vi "Get Arm Sensor Info.vi"(5 "error in (no error)":errorcluster, 6 "MotorControlDevRef":T1) -> (0 "error out":errorcluster, 1 "Current":dbl, 2 "Sensor Velocity":dbl, 3 "MotorControlDevRef out":T1, 4 "Sensor Position":dbl)   [LabVIEW 2020]
uses:
  <vilib>/Rock Robotics/WPI/MotorControl/WPI_MotorControlDeviceRef.ctl
  <vilib>/Rock Robotics/WPI/MotorControl/WPI_MotorControlType.ctl
  <vilib>/Rock Robotics/SystemInterfaces/DIO/FPGA_DIOPWMChannel.ctl
  <vilib>/Rock Robotics/WPI/PWM/WPI_PWMDeadband.ctl
  <vilib>/Rock Robotics/SystemInterfaces/DIO/FPGA_DIOChannel.ctl
  2023 Robot Global Data.vi
  <vilib>/Rock Robotics/Network Tables/NT Write Number.vi
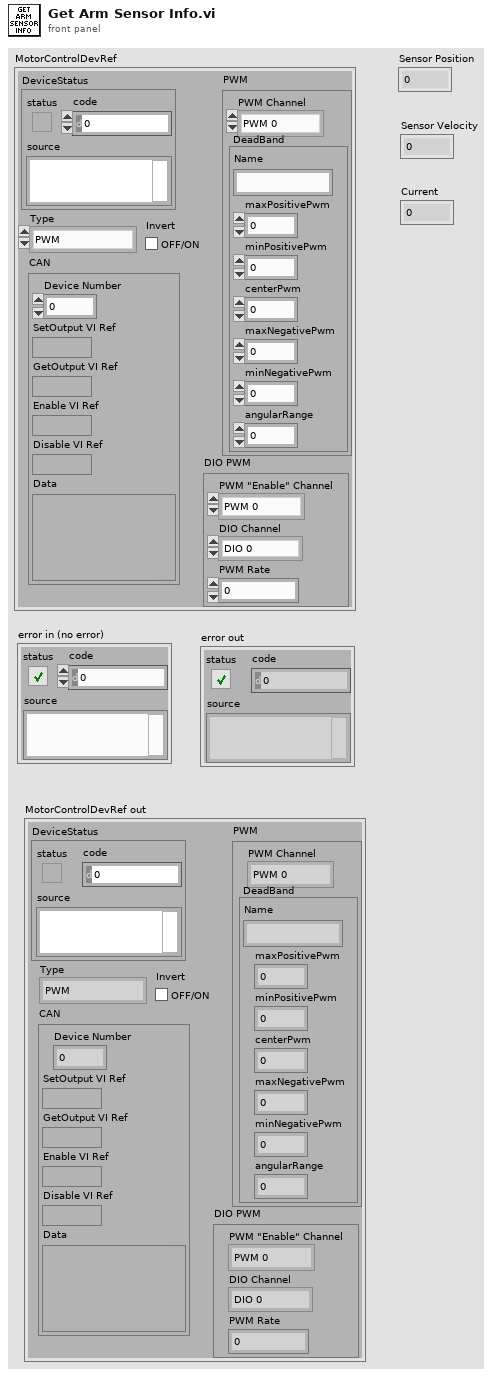
[diagram p1: front panel]
types:
  T1 = typedef "WPI_MotorControlDeviceRef.ctl" = cluster{"DeviceStatus":errorcluster, "Type":T2, "PWM":cluster{"PWM Channel":T3, "DeadBand":T4}, "CAN":cluster{"Device Number":u8, "SetOutput VI Ref":variant, "GetOutput VI Ref":variant, "Enable VI Ref":variant, "Disable VI Ref":variant, "Data":variant}, "Invert":bool, "DIO PWM":cluster{"PWM \"Enable\" Channel":T3, "DIOChannel":T5, "PWM Rate":dbl}}
  T2 = typedef "WPI_MotorControlType.ctl" = enum16{"PWM", "CAN", "DIO PWM"}
  T3 = typedef "FPGA_DIOPWMChannel.ctl" = enum8{"PWM 0", "PWM 1", "PWM 2", "PWM 3", "PWM 4", "PWM 5", "PWM 6", "PWM 7", "PWM 8", "PWM 9", "PWM MXP 0", "PWM MXP 1", "PWM MXP 2", "PWM MXP 3", "PWM MXP 4", "PWM MXP 5", "PWM MXP 6", "PWM MXP 7", "PWM MXP 8", "PWM MXP 9", "Invalid"}
  T4 = typedef "WPI_PWMDeadband.ctl" = cluster{"Name":string, "maxPositivePwm":i32, "minPositivePwm":i32, "centerPwm":i32, "maxNegativePwm":i32, "minNegativePwm":i32, "angularRange":u16}
  T5 = typedef "FPGA_DIOChannel.ctl" = enum8{"DIO 0", "DIO 1", "DIO 2", "DIO 3", "DIO 4", "DIO 5", "DIO 6", "DIO 7", "DIO 8", "DIO 9", "DIO MXP 0", "DIO MXP 1", "DIO MXP 2", "DIO MXP 3", "DIO MXP 4", "DIO MXP 5", "DIO MXP 6", "DIO MXP 7", "DIO MXP 8", "DIO MXP 9", "DIO MXP 10", "DIO MXP 11", "DIO MXP 12", "DIO MXP 13", "DIO MXP 14", "DIO MXP 15", "SPI Port CS1", "SPI Port CS2", "SPI Port CS3", "SPI Port MISO", "SPI Port MOSI", "Invalid"}
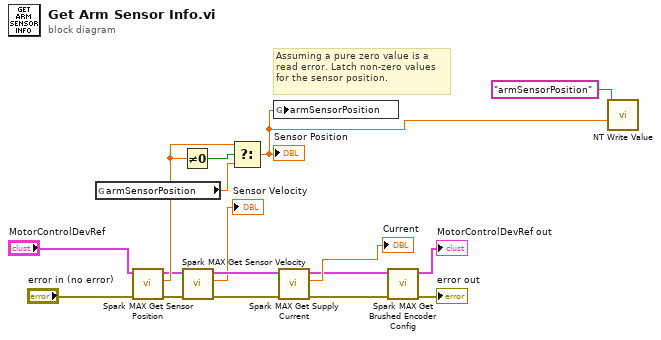
[diagram p0: block diagram]
diagram:
  # "Assuming a pure zero value is a\nread error. Latch non-zero values\nfor the sensor position."
  n1 = global read "2023 Robot Global Data.vi" "armSensorPosition"() -> (w8:dbl)
  n2 = call <vilib>:"Spark MAX Get Sensor Position.vi"("error in (no error)"="error in (no error)", "MotorControlDevRef in"="MotorControlDevRef") -> ("error out"=w3:errorcluster, "Sensor Position"=w5:dbl, "MotorControlDevRef out"=w4:T1)  [unwired: 6 in, 1 out]
  n3 = Not Equal To 0?(x=w5) -> (x != 0?=w9:bool)
  n4 = call <vilib>:"Spark MAX Get Sensor Velocity.vi"("error in (no error)"=w3, "MotorControlDevRef in"=w4) -> ("error out"=w16:errorcluster, "Sensor Velocity"=→"Sensor Velocity":dbl, "MotorControlDevRef out"=w15:T1)  [unwired: 6 in, 1 out]
  n5 = Select(t=w5, s=w9, f=w8) -> (s? t:f=w1:dbl)
  "Sensor Position" <- w1
  n6 = global write "2023 Robot Global Data.vi" "armSensorPosition"(w1) -> ()
  n7 = call <vilib>:"Spark MAX Get Supply Current.vi"("error in (no error)"=w16, "MotorControlDevRef in"=w15) -> ("error out"=w12:errorcluster, "Current"=→"Current":dbl, "MotorControlDevRef out"=w13:T1)  [unwired: 6 in, 1 out]
  n8 = call <vilib>:"Spark MAX Get Brushed Encoder Config.vi"("error in (no error)"=w12, "MotorControlDeviceRef in"=w13) -> ("error out"=→"error out":errorcluster, "MotorControlDeviceRef"=→"MotorControlDevRef out":T1)  [unwired: 4 in, 4 out]
  n9 = call-poly <vilib>:"NT Write Value.vi"("value"=w1, "name"="armSensorPosition") -> ()  [unwired: 9 in, 1 out]
